vi "Get Response.vi"(11 "Processing in":refnum<class "Processing.lvclass">) -> (2 "Response":refnum<class "Response.lvclass">, 3 "Processing out":refnum<class "Processing.lvclass">)   [LabVIEW 2020, in "HTTP Server.lvlib" / "Processing.lvclass"]
uses:
  Processing.lvclass
  Processing.lvclass/Processing.ctl
  lv-http-util/HTTP Utils/Response/Response.lvclass
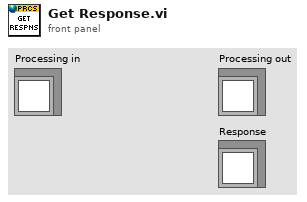
[diagram p1: front panel]
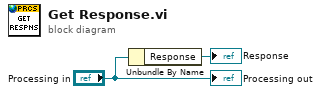
[diagram p0: block diagram]
diagram:
  n1 = Unbundle By Name("Processing in") -> ("Response"=→"Response":refnum<class "Response.lvclass">)
  "Processing out" <- "Processing in"
